vi "DeviceIDN.vi"(4 "error in (no error)":errorcluster, 6 "DeviceKey In":string, 7 "CmdLib In":refnum<k24>) -> (0 "error out":errorcluster, 1 "Response":string, 2 "DeviceKey Out":string, 3 "CmdLib Out":refnum<k24>)   [LabVIEW 2020]
uses:
  C:/GEECS/Developers Version/source/Device Drivers/Picomotor8742dotNet/NewFocus/CmdLib.dll
  NewFocus/CmdLib.dll
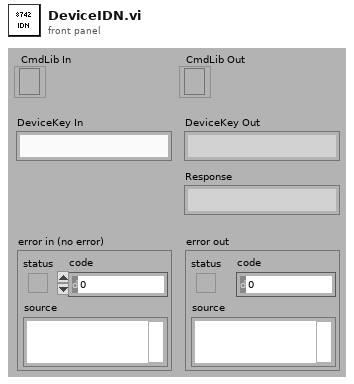
[diagram p1: front panel]
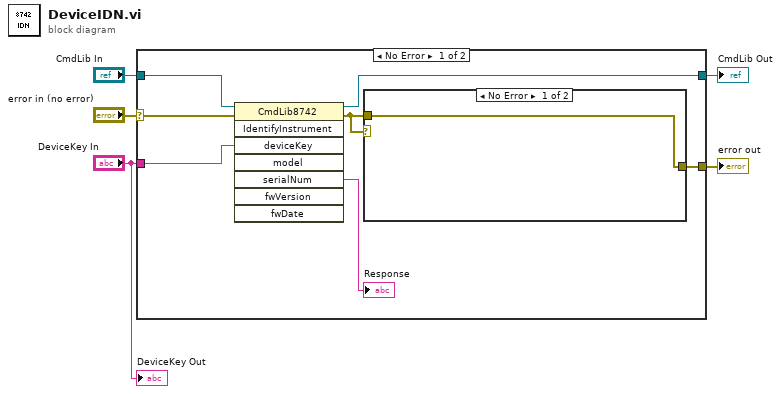
[diagram p0: block diagram]
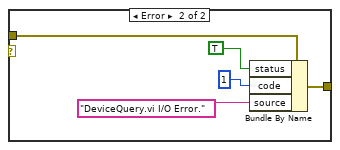
[diagram p2: hidden frame]
diagram:
  n1 = case shown="No Error" "error in (no error)" {
    selector: "error in (no error)" -> [w9 w20]
    tunnel: "CmdLib In" -> [w12 w19]
    tunnel: [w11 w19] -> w4
    tunnel: "DeviceKey In" -> [w10 _]
    tunnel: [w8 w20] -> w1
    frame No Error {
      n2 = invoke class="CmdLib8742" method="IdentifyInstrument"(reference=w12, error in=w9, "deviceKey"=w10) -> (reference out=w11:refnum<k24>, error out=w6:errorcluster, "serialNum"=→"Response":string)  [unwired: 5 in, 5 out]
      n3 = case shown="No Error" w6 {
        tunnel: w6 -> [w13 w16]
        tunnel: [w13 w15] -> w8
        frame No Error {
        }
        frame Error {
          n4 = Bundle By Name(cluster=w16, "status"=TRUE, "code"=1, "source"="DeviceQuery.vi I/O Error.") -> (w15:errorcluster)
        }
      }
    }
    frame Error {
    }
  }
  "CmdLib Out" <- w4
  "error out" <- w1
  "DeviceKey Out" <- "DeviceKey In"
